vi "Info Insert Row to 2D Int64 Array.vi"(5 "format string (%d)":string="%d", 6 "source info data":string, 7 "key description":string, 8 "sections in":string[](array[string]), 9 "row index to insert":i32, 10 "row to insert":i64[](array[numeric]), 11 "info data in":string) -> (0 "sections out":string[](array[string]), 3 "info data out":string)   [LabVIEW 2018]
doc: "Addition to infolib: Gets 2D array of int64 (if exits in the 'info data in'), inserts one row of int64 into it in selected row, writes it back."
uses:
  infolib.lvlibp/Private/Get matrix polymorph parts/Get 2D I64.vi
  infolib.lvlibp/Private/Add matrix polymorph parts/2D I64.vi
  infolib.lvlibp
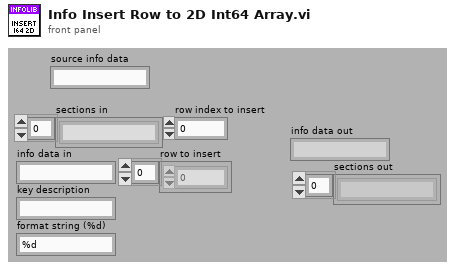
[diagram p1: front panel]
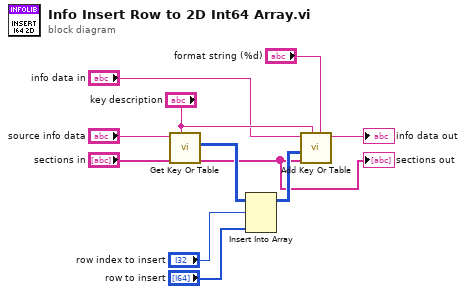
[diagram p0: block diagram]
diagram:
  n1 = call-poly "Get Key Or Table.vi"("key description"="key description", "sections"="sections in", "info data"="source info data") -> ("sections out"=w1:string[], "value"=w11:i64[][])  [unwired: 5 in, 2 out]
  "sections out" <- w1
  n2 = Insert Into Array(array=w11, index (row)="row index to insert", new element="row to insert") -> (w7:i64[][])  [unwired: 1 in]
  n3 = call-poly "Add Key Or Table.vi"("format string (%_20d)"="format string (%d)", "key description"="key description", "sections"=w1, "numeric"=w7, "info data"="info data in") -> ("info data out"=→"info data out":string)  [unwired: 6 in]
